vi "write_spectra_color_new_Flash.vi"() -> ()   [LabVIEW 2022 SP3]
uses:
  <vilib>/Utility/file.llb/Read From Spreadsheet File (DBL).vi
panel:
  in  "multiplied by":dbl=1.0
  out "second subarray":u8[](array[numeric])
  out "first subarray":u8[](array[numeric])
  out "size of array to write":i32
  out "Array to write":u8[](array[numeric])
  out "Waveform Graph 2":u16[](graph)
  in  "first row":dbl[](array[numeric])
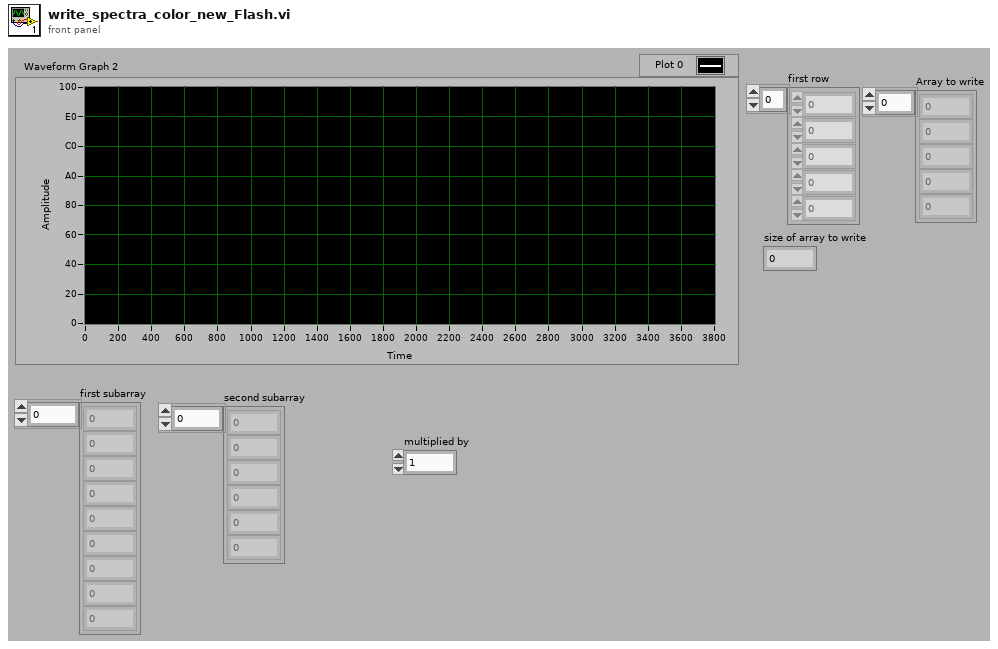
[diagram p1: front panel]
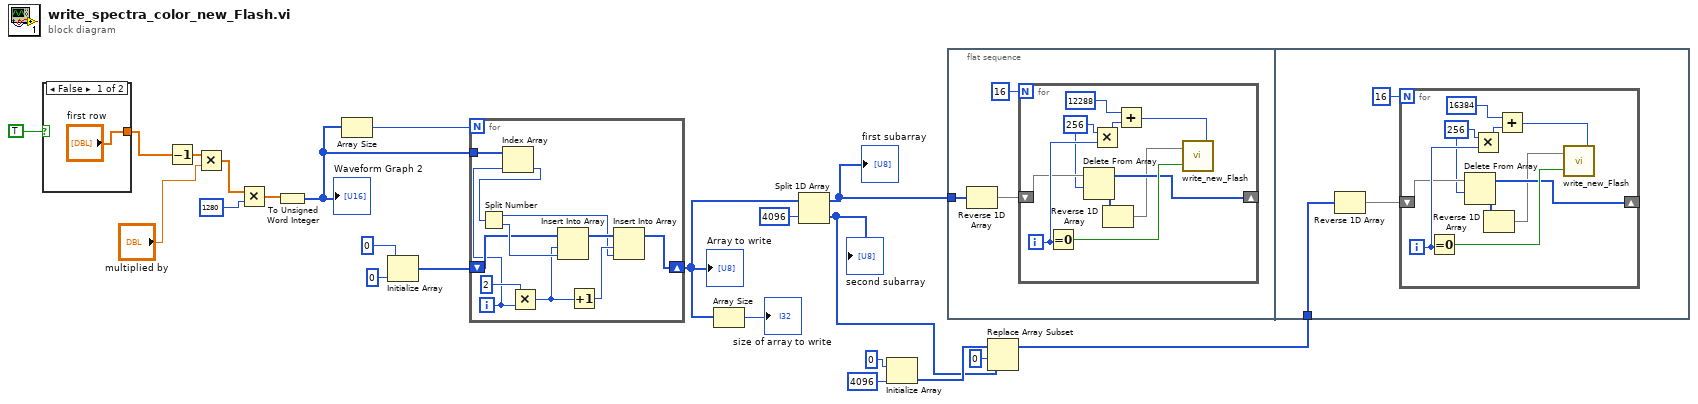
[diagram p0: block diagram]
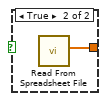
[diagram p2: hidden frame]
diagram:
  n1 = case shown="False" TRUE {
    tunnel: ["first row" w24] -> w4
    frame False {
    }
    frame True {
      n2 = call-poly <vilib>:"Read From Spreadsheet File.vi"() -> ("first row"=w24:dbl[])  [unwired: 7 in, 4 out]
    }
  }
  n3 = Decrement(x=w4) -> (x-1=w3:dbl[])
  n4 = Multiply(x=w3, y="multiplied by") -> (x*y=w1:dbl[])
  n5 = Multiply(x=w1, y=u16 1280) -> (x*y=w20:dbl[])
  n6 = To Unsigned Word Integer(number=w20) -> (unsigned 16bit integer=w19:u16[])
  "Waveform Graph 2" <- w19
  n7 = Array Size(array=w19) -> (size(s)=w14:i32)
  n8 = Initialize Array(u8 0 ("element"), 0 ("dimension size")) -> (w16:u8[])
  n9 = for {
    N: w14 -> [_]
    tunnel: w19 -> [w27]
    shift-right: [w28] -> w13
    shift-left: w16 -> [w33]
    i -> [w26]
    n10 = Index Array(array=w27, index=w26) -> (element=w25:u16)
    n11 = Split Number(x=w25) -> (hi(x)=w29:u8, lo(x)=w34:u8)
    n12 = Multiply(x=2, y=w26) -> (x*y=w31:i32)
    n13 = Insert Into Array(array=w33, index=w31, new element=w34) -> (w32:u8[])
    n14 = Increment(x=w31) -> (x+1=w30:i32)
    n15 = Insert Into Array(array=w32, index=w30, new element=w29) -> (w28:u8[])
  }
  "Array to write" <- w13
  n16 = Array Size(array=w13) -> (size(s)=→"size of array to write":i32)
  n17 = Split 1D Array(array=w13, index=4096) -> (first subarray=w11:u8[], second subarray=w7:u8[])
  "first subarray" <- w11
  "second subarray" <- w7
  n18 = Initialize Array(u8 0 ("element"), 4096 ("dimension size")) -> (w8:u8[])
  n19 = flat-sequence {
    tunnel: w11 -> [w37]
    tunnel: w6 -> [w49]
    frame #0 {
      n20 = Reverse 1D Array(array=w37) -> (reversed array=w36:u8[])
      n21 = for {
        N: 16 -> [_]
        shift-right: [w41] -> _
        shift-left: w36 -> [w44]
        i -> [w45]
        w43 = 256
        n22 = Equal To 0?(x=w45) -> (x = 0?=w48:bool)
        n23 = Delete From Array(array=w44, length=w43) -> (deleted portion=w40:u8[], array with subset deleted=w41:u8[])  [unwired: 1 in]
        n24 = Multiply(x=w43, y=w45) -> (x*y=w42:i32)
        n25 = Reverse 1D Array(array=w40) -> (reversed array=w39:u8[])
        n26 = Add(x=12288, y=w42) -> (x+y=w46:i32)
        n27 = call "write_new_Flash.vi"("address (3 bytes)"=w46, "sector erase"=w48, "write array"=w39) -> ()
      }
    }
    frame #1 {
      n28 = Reverse 1D Array(array=w49) -> (reversed array=w51:u8[])
      n29 = for {
        N: 16 -> [_]
        shift-right: [w54] -> _
        shift-left: w51 -> [w57]
        i -> [w58]
        w56 = 256
        n30 = Equal To 0?(x=w58) -> (x = 0?=w61:bool)
        n31 = Delete From Array(array=w57, length=w56) -> (deleted portion=w53:u8[], array with subset deleted=w54:u8[])  [unwired: 1 in]
        n32 = Multiply(x=w56, y=w58) -> (x*y=w55:i32)
        n33 = Reverse 1D Array(array=w53) -> (reversed array=w52:u8[])
        n34 = Add(x=16384, y=w55) -> (x+y=w59:i32)
        n35 = call "write_new_Flash.vi"("address (3 bytes)"=w59, "sector erase"=w61, "write array"=w52) -> ()
      }
    }
  }
  n36 = Replace Array Subset(array=w8, new element=w7, index=0) -> (w6:u8[])
